vi "test01.vi"() -> ()   [LabVIEW 2016, in "MB _relays.lvlib"]
uses:
  MB _relays.lvlib
  type defs/baudrate.ctl
  type defs/Relays IDs flash.ctl
  public/RELAYS Delayed OFF a Relay.vi
  public/RELAYS Delay ON a Relay.vi
  public/RELAYS Get Relay Status.vi
panel:
  out "ack 7":string
  out "Relay Status":bool[](array[boolean])
  in  "read relay status":bool
  out "success? 5":bool
  out "success? 4":bool
  out "success? 3":bool
  out "success? 2":bool
  out "success?":bool
  out "Written BD":T1=3 items=["4800"=2, "9600"=3, "19200"=4]
  out "Array":bool[](array[boolean])
  out "ack 6":string
  in  "Read optos":bool
  out "ack 5":string
  in  "Dev addr 2":u8=255
  in  "Write Dev Address":bool
  out "ack 4":string
  in  "Relays IDs 2":T2=3 items=["Relay 1"=3, "Relay 2"=8, "Relay 3"=13, "Relay 4"=18, "Relay 5"=23, "Relay 6"=28, "Relay 7"=33, "Relay 8"=38]
  out "ack 3":string
  in  "delayed Time (2 sec)":dbl
  in  "Relays IDs":T2=3 items=["Relay 1"=3, "Relay 2"=8, "Relay 3"=13, "Relay 4"=18, "Relay 5"=23, "Relay 6"=28, "Relay 7"=33, "Relay 8"=38]
  in  "flash ON":bool
  in  "flash OFF":bool
  out "ack 2":string
  in  "baudrate":T1=3 items=["4800"=2, "9600"=3, "19200"=4]
  out "ack":string
  in  "Write Baudrate":bool
  in  "Read Baudrate":bool
  out "Dev addr":u8=255
  in  "baud rate (19200)":u32=19200
  out "read buffer 3":string
  in  "ON OFF 2":bool
  in  "Turn all relays":bool
  in  "ON OFF":bool
  in  "Relay IDs":u16
  out "read buffer 2":string
  in  "Turn a Relay":bool
  in  "Clear":bool
  in  "VISA resource name":refnum<visa-resource-name>="COM3"
  out "read buffer":string
  in  "Read Dev Address":bool
  in  "stop":bool
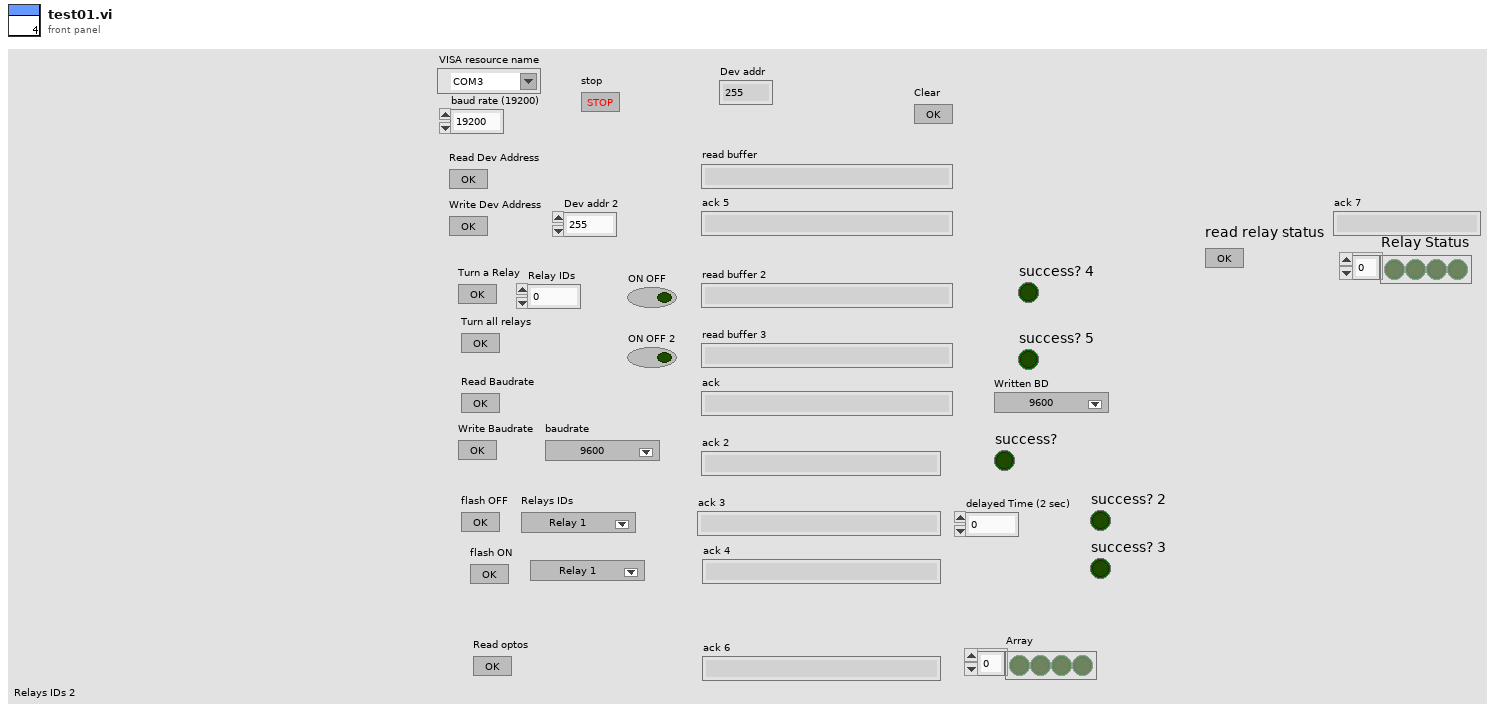
[diagram p1: front panel]
types:
  T1 = typedef "MB _relays.lvlib/baudrate.ctl" = u8
  T2 = typedef "MB _relays.lvlib/Relays IDs flash.ctl" = u16
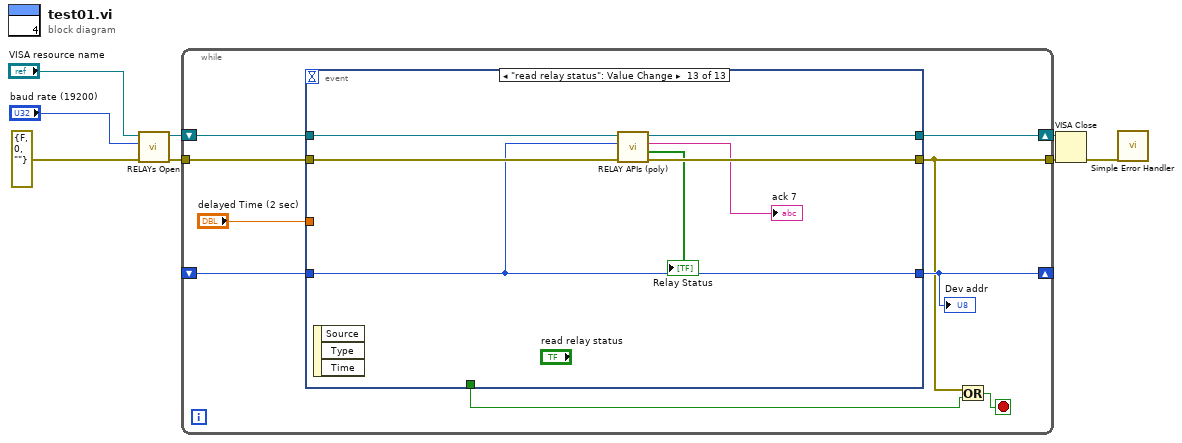
[diagram p0: block diagram]
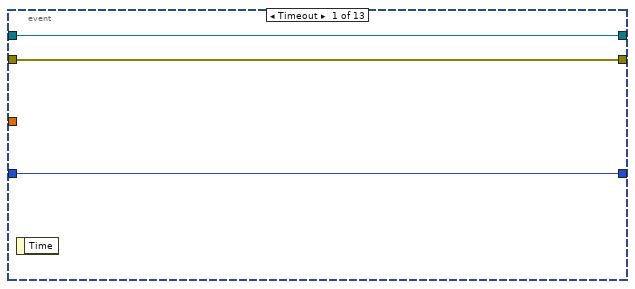
[diagram p2: hidden frame]
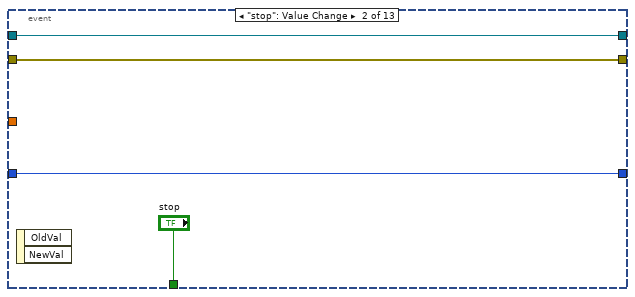
[diagram p3: hidden frame]
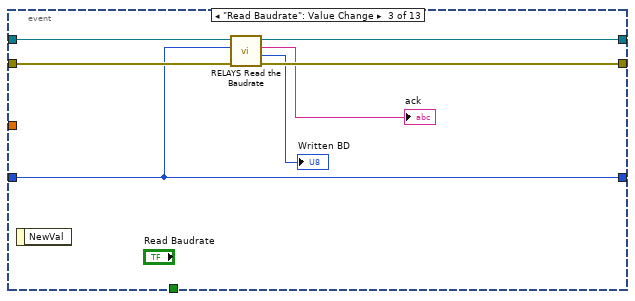
[diagram p4: hidden frame]
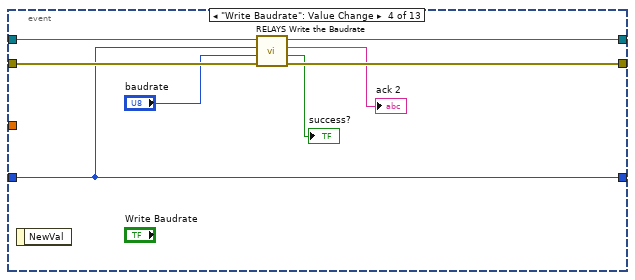
[diagram p5: hidden frame]
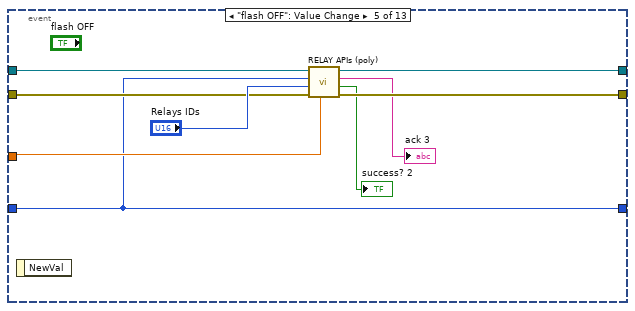
[diagram p6: hidden frame]
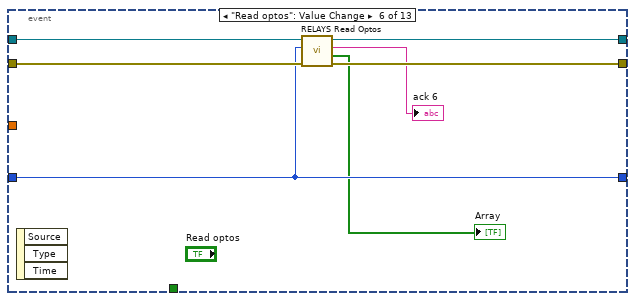
[diagram p7: hidden frame]
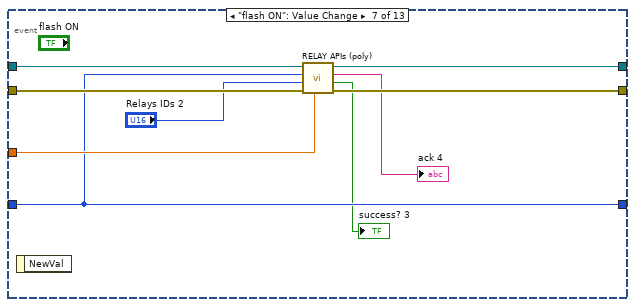
[diagram p8: hidden frame]
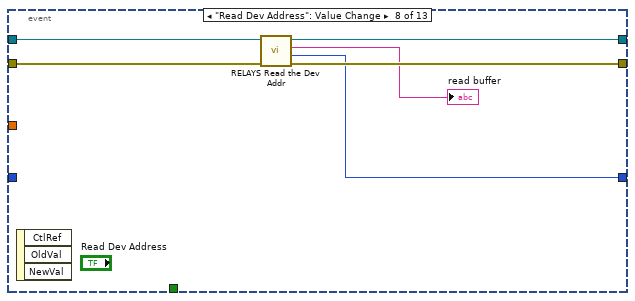
[diagram p9: hidden frame]
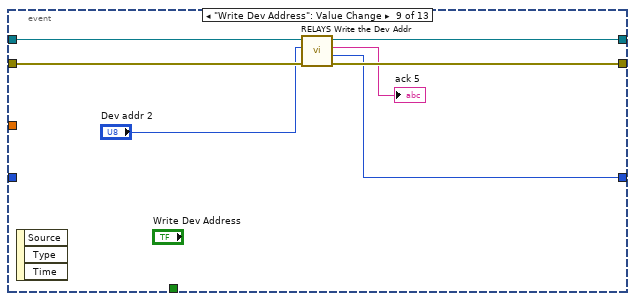
[diagram p10: hidden frame]
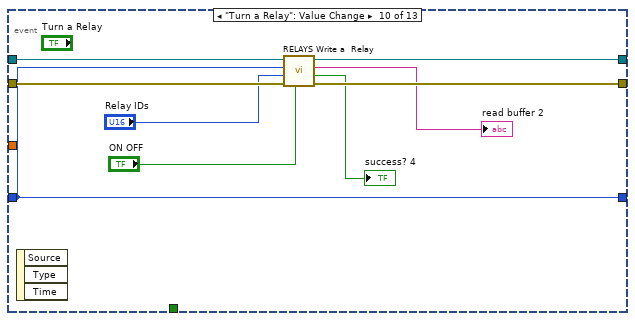
[diagram p11: hidden frame]
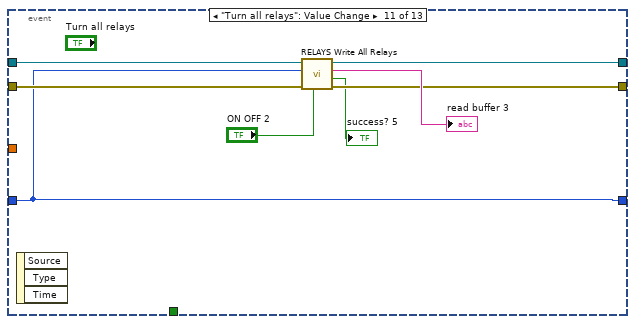
[diagram p12: hidden frame]
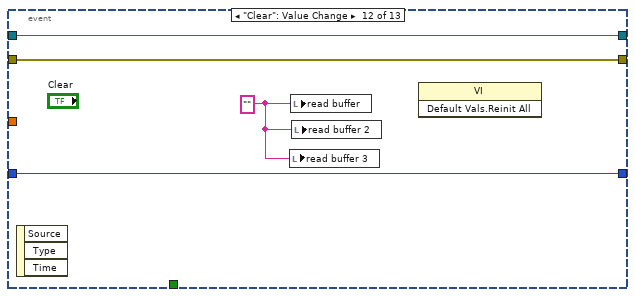
[diagram p13: hidden frame]
diagram:
  n1 = call "RELAYs Open.vi"("error in (no error)"=errorcluster {"status"=FALSE, "code"=0, "source"=""}, "baud rate (19200)"="baud rate (19200)", "VISA resource name"="VISA resource name") -> ("error out"=w5:errorcluster, "VISA resource name out"=w6:refnum<visa-resource-name>)  [unwired: 7 in]
  n2 = while {
    tunnel: w5 -> [w17]
    tunnel: [w9] -> w3
    shift-right: [w15] -> w4
    shift-left: w6 -> [w16]
    shift-right: [w13] -> _
    shift-left: _ -> [w12]
    stop <- w10 stop-if-true
    n3 = event shown="[12] \"read relay status\": Value Change" {
      selector: _ -> [_ _ _ _ _ _ _ _ _ _ _ _ _]
      dyn-events: _ -> [_ _ _ _ _ _ _ _ _ _ _ _ _]
      timeout: _ -> [_ _ _ _ _ _ _ _ _ _ _ _ _]
      tunnel: [_ "stop" _ _ _ _ _ _ _ _ _ _ _] -> w11
      tunnel: w17 -> [w19 w22 w29 w37 w46 w55 w62 w69 w77 w85 w92 w97 w104]
      tunnel: w16 -> [w20 w23 w31 w39 w48 w53 w64 w70 w75 w86 w94 w98 w105]
      tunnel: [w20 w23 w30 w38 w45 w52 w63 w68 w74 w81 w89 w98 w103] -> w15
      tunnel: [w19 w22 w28 w36 w44 w54 w61 w67 w76 w82 w90 w97 w102] -> w9
      tunnel: "delayed Time (2 sec)" -> [_ _ _ _ w42 _ w58 _ _ _ _ _ _]
      tunnel: [w18 w21 w26 w33 w41 w51 w57 w65 w71 w79 w88 w95 w101] -> w13
      tunnel: w12 -> [w18 w21 w26 w33 w41 w51 w57 _ _ w79 w88 w95 w101]
      event Timeout {
        n4 = event-data() -> ()  [unwired: 1 in, 1 out]
      }
      event "stop": Value Change {
        n5 = event-data() -> ()  [unwired: 1 in, 2 out]
      }
      event "Read Baudrate": Value Change {
        n6 = event-data() -> ()  [unwired: 1 in, 1 out]
        n7 = call "RELAYS Read the Baudrate.vi"("error in (no error)"=w29, "Dev addr"=w26, "VISA resource name"=w31) -> ("error out"=w28:errorcluster, "baudrate"=→"Written BD":T1, "ack"=→"ack":string, "VISA resource name out"=w30:refnum<visa-resource-name>)  [unwired: 5 in]
      }
      event "Write Baudrate": Value Change {
        n8 = event-data() -> ()  [unwired: 1 in, 1 out]
        n9 = call "RELAYS Write the Baudrate.vi"("error in (no error)"=w37, "baudrate"="baudrate", "Dev addr"=w33, "VISA resource name"=w39) -> ("error out"=w36:errorcluster, "success?"=→"success?":bool, "ack"=→"ack 2":string, "VISA resource name out"=w38:refnum<visa-resource-name>)  [unwired: 4 in]
      }
      event "flash OFF": Value Change {
        n10 = event-data() -> ()  [unwired: 1 in, 1 out]
        n11 = call-poly "RELAY APIs (poly).vi"("Delayed Time( 2 sec)"=w42, "error in (no error)"=w46, "Relays IDs"="Relays IDs", "Dev addr"=w41, "VISA resource name"=w48) -> ("error out"=w44:errorcluster, "success?"=→"success? 2":bool, "ack"=→"ack 3":string, "VISA resource name out"=w45:refnum<visa-resource-name>)  [unwired: 3 in]
      }
      event "Read optos": Value Change {
        n12 = event-data() -> ()  [unwired: 1 in, 3 out]
        n13 = call "RELAYS Read Optos.vi"("error in (no error)"=w55, "Dev Addr"=w51, "VISA resource name"=w53) -> ("error out"=w54:errorcluster, "Optos Status"=→"Array":bool[], "ack"=→"ack 6":string, "VISA resource name out"=w52:refnum<visa-resource-name>)  [unwired: 5 in]
      }
      event "flash ON": Value Change {
        n14 = event-data() -> ()  [unwired: 1 in, 1 out]
        n15 = call-poly "RELAY APIs (poly).vi"("delayed Time ( 2 sec)"=w58, "error in (no error)"=w62, "Relays IDs"="Relays IDs 2", "Dev addr"=w57, "VISA resource name"=w64) -> ("error out"=w61:errorcluster, "success?"=→"success? 3":bool, "ack"=→"ack 4":string, "VISA resource name out"=w63:refnum<visa-resource-name>)  [unwired: 3 in]
      }
      event "Read Dev Address": Value Change {
        n16 = event-data() -> ()  [unwired: 1 in, 3 out]
        n17 = call "RELAYS Read the Dev Addr.vi"("error in (no error)"=w69, "VISA resource name"=w70) -> ("error out"=w67:errorcluster, "Dev Address"=w65:u8, "ack"=→"read buffer":string, "VISA resource name out"=w68:refnum<visa-resource-name>)  [unwired: 6 in]
      }
      event "Write Dev Address": Value Change {
        n18 = event-data() -> ()  [unwired: 1 in, 3 out]
        n19 = call "RELAYS Write the Dev Addr.vi"("error in (no error)"=w77, "Dev Addr"="Dev addr 2", "VISA resource name"=w75) -> ("error out"=w76:errorcluster, "written Address"=w71:u8, "ack"=→"ack 5":string, "VISA resource name out"=w74:refnum<visa-resource-name>)  [unwired: 5 in]
      }
      event "Turn a Relay": Value Change {
        n20 = event-data() -> ()  [unwired: 1 in, 3 out]
        n21 = call "RELAYS Write a  Relay.vi"("ON OFF"="ON OFF", "error in (no error)"=w85, "Relay IDs"="Relay IDs", "Dev addr"=w79, "VISA resource name"=w86) -> ("error out"=w82:errorcluster, "success?"=→"success? 4":bool, "ack"=→"read buffer 2":string, "VISA resource name out"=w81:refnum<visa-resource-name>)  [unwired: 3 in]
      }
      event "Turn all relays": Value Change {
        n22 = event-data() -> ()  [unwired: 1 in, 3 out]
        n23 = call "RELAYS Write All Relays.vi"("ON_OFF"="ON OFF 2", "error in (no error)"=w92, "Dev addr"=w88, "VISA resource name"=w94) -> ("error out"=w90:errorcluster, "success?"=→"success? 5":bool, "ack"=→"read buffer 3":string, "VISA resource name out"=w89:refnum<visa-resource-name>)  [unwired: 4 in]
      }
      event "Clear": Value Change {
        w96 = "" ("read buffer")
        n24 = event-data() -> ()  [unwired: 1 in, 3 out]
        n25 = local write "read buffer 3"(w96) -> ()
        n26 = local write "read buffer"(w96) -> ()
        n27 = local write "read buffer 2"(w96) -> ()
        n28 = invoke class="VI" method="Default Vals.Reinit All"() -> ()  [unwired: 3 in, 3 out]
      }
      event "read relay status": Value Change {
        n29 = event-data() -> ()  [unwired: 1 in, 3 out]
        n30 = call-poly "RELAY APIs (poly).vi"("error in (no error)"=w104, "Dev addr"=w101, "VISA resource name"=w105) -> ("error out"=w102:errorcluster, "Relay Status"=→"Relay Status":bool[], "ack"=→"ack 7":string, "VISA resource name out"=w103:refnum<visa-resource-name>)  [unwired: 5 in]
      }
    }
    "Dev addr" <- w13
    n31 = Or(x=w9, y=w11) -> (x .or. y?=w10:bool)
  }
  n32 = VISA Close(VISA resource name=w4, error in (no error)=w3) -> (error out=w2:errorcluster)
  n33 = call <vilib>:"Simple Error Handler.vi"("error in (no error)"=w2) -> ()  [unwired: 4 in, 5 out]
